vi "HP1200_009_ack_error.vi"(7 "device_addr":u16=22, 8 "error in":errorcluster, 11 "conn_id_in":refnum<k5>) -> (0 "error out":errorcluster, 1 "response":string, 2 "ack_ok":bool=TRUE, 3 "conn_id_out":refnum<k5>, 4 "status":bool, 5 "ack_ret":string)   [LabVIEW 2019]
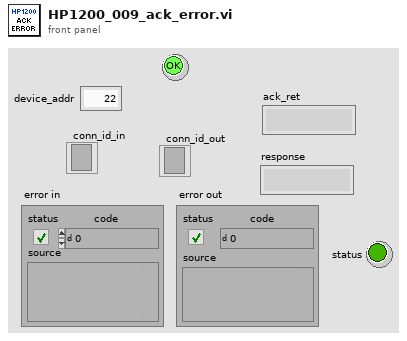
[diagram p1: front panel]
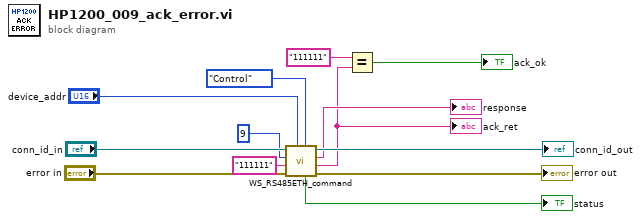
[diagram p0: block diagram]
diagram:
  n1 = call "WS_RS485ETH_command.vi"("action"=enum16{"Request", "Control"}."Control", "device_addr"="device_addr", "error in"="error in", "data_string"="111111", "param_num"=u16 9, "conn_id_in"="conn_id_in") -> ("error out"=→"error out":errorcluster, "data_out"=w3:string, "response"=→"response":string, "conn_id_out"=→"conn_id_out":refnum<k5>, "status"=→"status":bool)  [unwired: 1 in]
  "ack_ret" <- w3
  n2 = Equal?(x="111111", y=w3) -> (x = y?=→"ack_ok":bool)
